vi "test-rotation3d.vi"(8 "error in (no error)":errorcluster) -> (0 "error out":errorcluster, 3 "ALL TESTS PASSED":bool)   [LabVIEW 2019]
uses:
  <vilib>/Rock Robotics/WPI/ThirdParty/JAS_Junk/TrajLib/Quaternion_New_Default.vi
  <vilib>/Rock Robotics/WPI/ThirdParty/JAS_Junk/TrajLib/Matrix_NormF.vi
  <vilib>/Rock Robotics/WPI/ThirdParty/JAS_Junk/TrajLib/Quaternion_New.vi
  <vilib>/Rock Robotics/WPI/ThirdParty/JAS_Junk/TrajLib/Rotation3d_Times.vi
  <vilib>/Rock Robotics/WPI/ThirdParty/JAS_Junk/TrajLib/MathUtil_Clamp.vi
  <vilib>/Rock Robotics/WPI/ThirdParty/JAS_Junk/TrajLib/Quaternion_Get_All.vi
  <vilib>/Rock Robotics/WPI/ThirdParty/JAS_Junk/TrajLib/Rotation3d_GetQuaterion.vi
  <vilib>/Rock Robotics/WPI/ThirdParty/JAS_Junk/TrajLib/Quaternion_Equals.vi
  <vilib>/Rock Robotics/WPI/ThirdParty/JAS_Junk/TrajLib/Util_CalcDist.vi
  <vilib>/Rock Robotics/WPI/ThirdParty/JAS_Junk/TrajLib/Quaternion_Get_Vect.vi
  <vilib>/Rock Robotics/WPI/ThirdParty/JAS_Junk/TrajLib/Quaternion_Get_W.vi
  <vilib>/Rock Robotics/WPI/ThirdParty/JAS_Junk/TrajLib/Rotation3d_UnaryMinus.vi
  <vilib>/Rock Robotics/WPI/ThirdParty/JAS_Junk/TrajLib/Rotation3d_Create_Quaternion.vi
  <vilib>/Rock Robotics/WPI/ThirdParty/JAS_Junk/TrajLib/Quaternion_Times.vi
  <vilib>/Analysis/_algsub.llb/Matrix Norm.vi
  <vilib>/Analysis/_algsub.llb/Real Matrix Norm.vi
  <vilib>/Rock Robotics/WPI/ThirdParty/JAS_Junk/TrajLib/Quaternion_Inverse.vi
  <vilib>/Rock Robotics/WPI/ThirdParty/JAS_Junk/TrajLib/Quaternion_Normalize.vi
  <vilib>/Rock Robotics/WPI/ThirdParty/JAS_Junk/TrajLib/Quaternion_Get_LVQuat.vi
  <vilib>/Rock Robotics/WPI/ThirdParty/JAS_Junk/TrajLib/Quaternion_New_LVQuat.vi
  <vilib>/Analysis/Matrix/Numeric/Conversions/Array To Matrix - RA.vi
  <vilib>/robotics/Kinematics/Multiply Quaternions.vi
  <vilib>/robotics/Kinematics/Multiply Quaternion by Quaternion.vi
  <vilib>/Rock Robotics/WPI/ThirdParty/JAS_Junk/TrajLib/Trajectory_Library.lvlib
  <vilib>/Analysis/Matrix/NI_Matrix.lvlib
panel:
  # "ROTATION3D TEST"
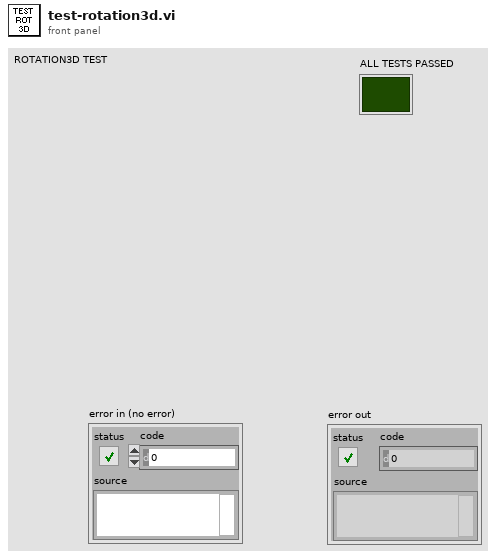
[diagram p1: front panel]
types:
  T1 = typedef "Trajectory_Library.lvlib/ROTATION3D.ctl" = cluster{"Q_quaternion":T2}
  T2 = typedef "Trajectory_Library.lvlib/QUATERNION.ctl" = cluster{"R":dbl, "V":dbl[]}
  T3 = typedef "Trajectory_Library.lvlib/ROTATION2D.ctl" = cluster{"VALUE":dbl, "COS":dbl, "SIN":dbl}
  T4 = typedef "NI_Matrix.lvlib/RealMatrix.ctl" = dbl[][]
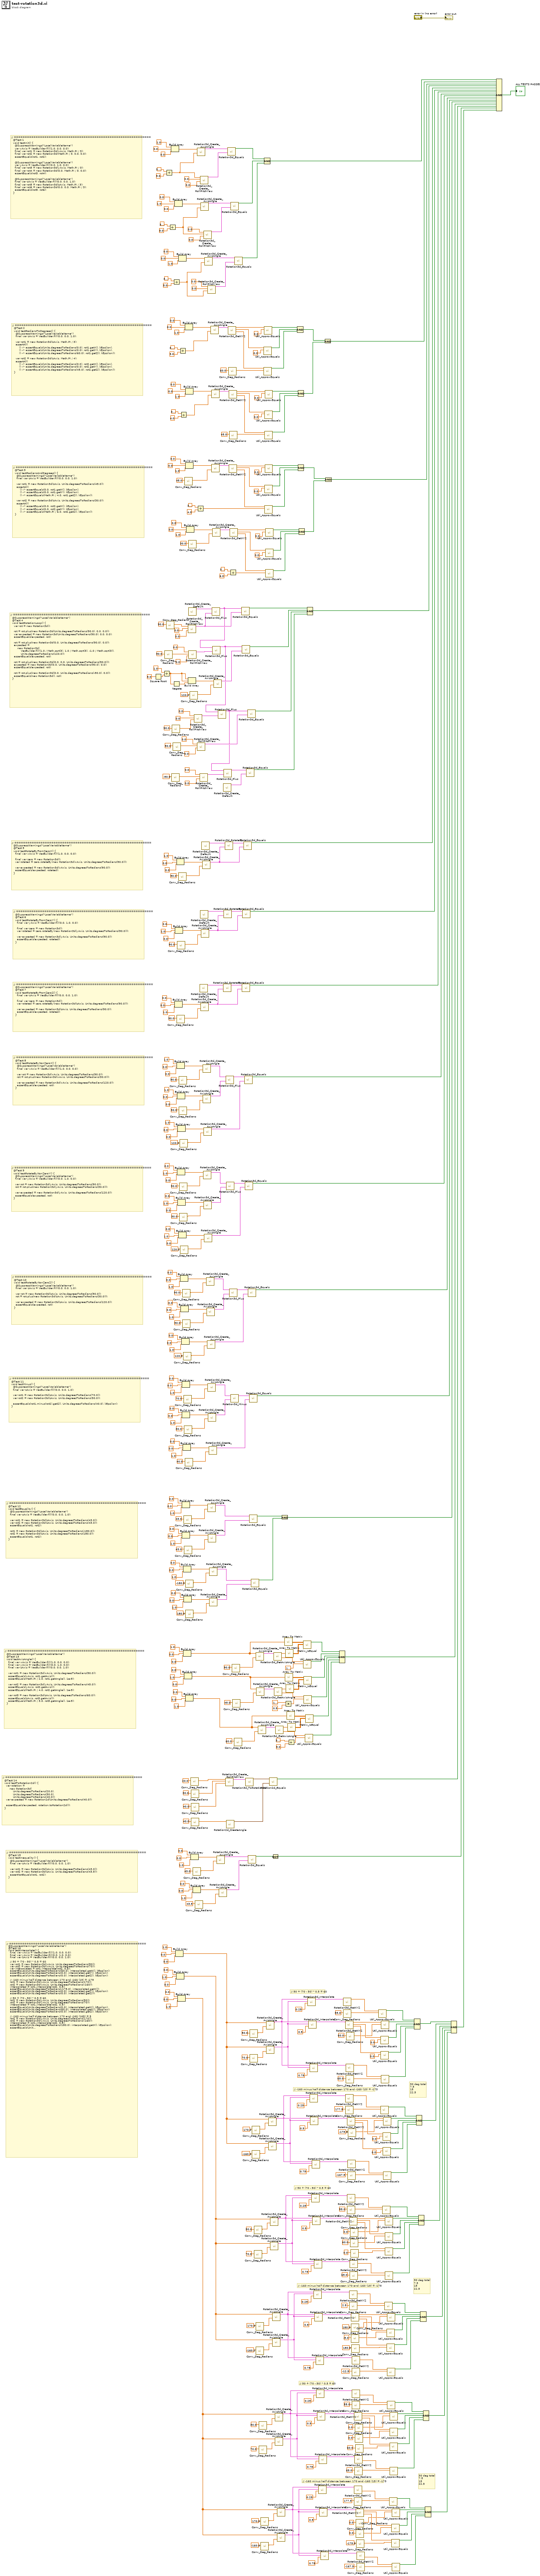
[diagram p0: block diagram]
diagram:
  # "30 deg total\n7.5\n15\n22.5"
  # "// -160 minus half distance between 170 and -160 (15) = -175"
  # "// 50 + (70 - 50) * 0.5 = 60"
  # "30 deg total\n7.5\n15\n22.5"
  # "// -160 minus half distance between 170 and -160 (15) = -175"
  # "// 50 + (70 - 50) * 0.5 = 60"
  # "30 deg total\n7.5\n15\n22.5"
  # "// -160 minus half distance between 170 and -160 (15) = -175"
  # "// 50 + (70 - 50) * 0.5 = 60"
  # "// ===============================================================\n  @SuppressWarnings(\"LocalVariableName\")\n  @Test 16\n  void testInterpolate() {\n    final var xAxis = VecBuilder.fill(1.0, 0.0, 0.0);\n    final var yAxis = VecBuilder.fill(0.0, 1.0, 0.0);\n    final var zAxis = VecBuilder.fill(0.0, 0.0, 1.0);\n\n    // 50 + (70 - 50) * 0.5 = 60\n    var rot1 = new Rotation3d(xAxis, Units.degreesToRadians(50));\n    var rot2 = new Rotation3d(xAxis, Units.degreesToRadians(70));\n    var interpolated = rot1.interpolate(rot2, 0.5);\n    assertEquals(Units.degreesToRadians(60.0), interpolated.getX(), kEpsilon);\n    assertEquals(Units.degreesToRadians(0.0), interpolated.getY(), kEpsilon);\n    assertEquals(Units.degreesToRadians(0.0), interpolated.getZ(), kEpsilon);\n\n    // -160 minus half distance between 170 and -160 (15) = -175\n    rot1 = new Rotation3d(xAxis, Units.degreesToRadians(170));\n    rot2 = new Rotation3d(xAxis, Units.degreesToRadians(-160));\n    interpolated = rot1.interpolate(rot2, 0.5);\n    assertEquals(Units.degreesToRadians(-175.0), interpolated.getX());\n    assertEquals(Units.degreesToRadians(0.0), interpolated.getY(), kEpsilon);\n    assertEquals(Units.degreesToRadians(0.0), interpolated.getZ());\n\n    // 50 + (70 - 50) * 0.5 = 60\n    rot1 = new Rotation3d(yAxis, Units.degreesToRadians(50));\n    rot2 = new Rotation3d(yAxis, Units.degreesToRadians(70));\n    interpolated = rot1.interpolate(rot2, 0.5);\n    assertEquals(Units.degreesToRadians(0.0), interpolated.getX(), kEpsilon);\n    assertEquals(Units.degreesToRadians(60.0), interpolated.getY(), kEpsilon);\n    assertEquals(Units.degreesToRadians(0.0), interpolated.getZ(), kEpsilon);\n\n    // -160 minus half distance between 170 and -160 (165) = 5\n    rot1 = new Rotation3d(yAxis, Units.degreesToRadians(170));\n    rot2 = new Rotation3d(yAxis, Units.degreesToRadians(-160));\n    interpolated = rot1.interpolate(rot2, 0.5);\n    assertEquals(Units.degreesToRadians(180.0), interpolated.getX(), kEpsilon);\n    assertEquals(Units.degreesToRadians(-5.0), interpolated.getY(), kEpsilon);\n    assertEquals(Units.degreesToRadians(180.0), interpolated.getZ(), kEpsilon);\n\n    // 50 + (70 - 50) * 0.5 = 60\n    rot1 = new Rotation3d(zAxis, Units.degreesToRadians(50));\n    rot2 = new Rotation3d(zAxis, Units.degreesToRadians(70));\n    interpolated = rot1.interpolate(rot2, 0.5);\n    assertEquals(Units.degreesToRadians(0.0), interpolated.getX(), kEpsilon);\n    assertEquals(Units.degreesToRadians(0.0), interpolated.getY(), kEpsilon);\n    assertEquals(Units.degreesToRadians(60.0), interpolated.getZ(), kEpsilon);\n\n    // -160 minus half distance between 170 and -160 (15) = -175\n    rot1 = new Rotation3d(zAxis, Units.degreesToRadians(170));\n    rot2 = new Rotation3d(zAxis, Units.degreesToRadians(-160));\n    interpolated = rot1.interpolate(rot2, 0.5);\n    assertEquals(Units.degreesToRadians(0.0), interpolated.getX(), kEpsilon);\n    assertEquals(Units.degreesToRadians(0.0), interpolated.getY(), kEpsilon);\n    assertEquals(Units.degreesToRadians(-175.0), interpolated.getZ(), kEpsilon);\n  }"
  # "// ===============================================================\n  @Test 15\n  void testInequality() {\n    @SuppressWarnings(\"LocalVariableName\")\n    final var zAxis = VecBuilder.fill(0.0, 0.0, 1.0);\n\n    var rot1 = new Rotation3d(zAxis, Units.degreesToRadians(43.0));\n    var rot2 = new Rotation3d(zAxis, Units.degreesToRadians(43.5));\n    assertNotEquals(rot1, rot2);\n  }"
  # "// ===============================================================\n  @Test 14\n  void testToRotation2d() {\n    var rotation =\n        new Rotation3d(\n            Units.degreesToRadians(20.0),\n            Units.degreesToRadians(30.0),\n            Units.degreesToRadians(40.0));\n    var expected = new Rotation2d(Units.degreesToRadians(40.0));\n\n    assertEquals(expected, rotation.toRotation2d());\n  }"
  # "// ===============================================================\n  @SuppressWarnings(\"LocalVariableName\")\n  @Test 13\n  void testAxisAngle() {\n    final var xAxis = VecBuilder.fill(1.0, 0.0, 0.0);\n    final var yAxis = VecBuilder.fill(0.0, 1.0, 0.0);\n    final var zAxis = VecBuilder.fill(0.0, 0.0, 1.0);\n\n    var rot1 = new Rotation3d(xAxis, Units.degreesToRadians(90.0));\n    assertEquals(xAxis, rot1.getAxis());\n    assertEquals(Math.PI / 2.0, rot1.getAngle(), 1e-9);\n\n    var rot2 = new Rotation3d(yAxis, Units.degreesToRadians(45.0));\n    assertEquals(yAxis, rot2.getAxis());\n    assertEquals(Math.PI / 4.0, rot2.getAngle(), 1e-9);\n\n    var rot3 = new Rotation3d(zAxis, Units.degreesToRadians(60.0));\n    assertEquals(zAxis, rot3.getAxis());\n    assertEquals(Math.PI / 3.0, rot3.getAngle(), 1e-9);\n  }"
  # "// ===============================================================\n  @Test 12\n  void testEquality() {\n    @SuppressWarnings(\"LocalVariableName\")\n    final var zAxis = VecBuilder.fill(0.0, 0.0, 1.0);\n\n    var rot1 = new Rotation3d(zAxis, Units.degreesToRadians(43.0));\n    var rot2 = new Rotation3d(zAxis, Units.degreesToRadians(43.0));\n    assertEquals(rot1, rot2);\n\n    rot1 = new Rotation3d(zAxis, Units.degreesToRadians(-180.0));\n    rot2 = new Rotation3d(zAxis, Units.degreesToRadians(180.0));\n    assertEquals(rot1, rot2);\n  }"
  # "// ===============================================================\n  @Test 11\n  void testMinus() {\n    @SuppressWarnings(\"LocalVariableName\")\n    final var zAxis = VecBuilder.fill(0.0, 0.0, 1.0);\n\n    var rot1 = new Rotation3d(zAxis, Units.degreesToRadians(70.0));\n    var rot2 = new Rotation3d(zAxis, Units.degreesToRadians(30.0));\n\n    assertEquals(rot1.minus(rot2).getZ(), Units.degreesToRadians(40.0), kEpsilon);\n  }"
  # "// ===============================================================\n  @Test 10\n  void testRotateByNonZeroZ() {\n    @SuppressWarnings(\"LocalVariableName\")\n    final var zAxis = VecBuilder.fill(0.0, 0.0, 1.0);\n\n    var rot = new Rotation3d(zAxis, Units.degreesToRadians(90.0));\n    rot = rot.plus(new Rotation3d(zAxis, Units.degreesToRadians(30.0)));\n\n    var expected = new Rotation3d(zAxis, Units.degreesToRadians(120.0));\n    assertEquals(expected, rot);\n  }"
  # "// ===============================================================\n  @Test 9\n  void testRotateByNonZeroY() {\n    @SuppressWarnings(\"LocalVariableName\")\n    final var yAxis = VecBuilder.fill(0.0, 1.0, 0.0);\n\n    var rot = new Rotation3d(yAxis, Units.degreesToRadians(90.0));\n    rot = rot.plus(new Rotation3d(yAxis, Units.degreesToRadians(30.0)));\n\n    var expected = new Rotation3d(yAxis, Units.degreesToRadians(120.0));\n    assertEquals(expected, rot);\n  }"
  # "// ===============================================================\n  @Test 8\n  void testRotateByNonZeroX() {\n    @SuppressWarnings(\"LocalVariableName\")\n    final var xAxis = VecBuilder.fill(1.0, 0.0, 0.0);\n\n    var rot = new Rotation3d(xAxis, Units.degreesToRadians(90.0));\n    rot = rot.plus(new Rotation3d(xAxis, Units.degreesToRadians(30.0)));\n\n    var expected = new Rotation3d(xAxis, Units.degreesToRadians(120.0));\n    assertEquals(expected, rot);\n  }"
  # "// ===============================================================\n  @SuppressWarnings(\"LocalVariableName\")\n  @Test 7\n  void testRotateByFromZeroZ() {\n    final var zAxis = VecBuilder.fill(0.0, 0.0, 1.0);\n\n    final var zero = new Rotation3d();\n    var rotated = zero.rotateBy(new Rotation3d(zAxis, Units.degreesToRadians(90.0)));\n\n    var expected = new Rotation3d(zAxis, Units.degreesToRadians(90.0));\n    assertEquals(expected, rotated);\n  }"
  # "// ===============================================================\n  @SuppressWarnings(\"LocalVariableName\")\n  @Test 6\n  void testRotateByFromZeroY() {\n    final var yAxis = VecBuilder.fill(0.0, 1.0, 0.0);\n\n    final var zero = new Rotation3d();\n    var rotated = zero.rotateBy(new Rotation3d(yAxis, Units.degreesToRadians(90.0)));\n\n    var expected = new Rotation3d(yAxis, Units.degreesToRadians(90.0));\n    assertEquals(expected, rotated);\n  }"
  # "// ===============================================================\n  @SuppressWarnings(\"LocalVariableName\")\n  @Test 5\n  void testRotateByFromZeroX() {\n    final var xAxis = VecBuilder.fill(1.0, 0.0, 0.0);\n\n    final var zero = new Rotation3d();\n    var rotated = zero.rotateBy(new Rotation3d(xAxis, Units.degreesToRadians(90.0)));\n\n    var expected = new Rotation3d(xAxis, Units.degreesToRadians(90.0));\n    assertEquals(expected, rotated);\n  }"
  # "// ===============================================================\n  @SuppressWarnings(\"LocalVariableName\")\n  @Test 4\n  void testRotationLoop() {\n    var rot = new Rotation3d();\n\n    rot = rot.plus(new Rotation3d(Units.degreesToRadians(90.0), 0.0, 0.0));\n    var expected = new Rotation3d(Units.degreesToRadians(90.0), 0.0, 0.0);\n    assertEquals(expected, rot);\n\n    rot = rot.plus(new Rotation3d(0.0, Units.degreesToRadians(90.0), 0.0));\n    expected =\n        new Rotation3d(\n            VecBuilder.fill(1.0 / Math.sqrt(3), 1.0 / Math.sqrt(3), -1.0 / Math.sqrt(3)),\n            Units.degreesToRadians(120.0));\n    assertEquals(expected, rot);\n\n    rot = rot.plus(new Rotation3d(0.0, 0.0, Units.degreesToRadians(90.0)));\n    expected = new Rotation3d(0.0, Units.degreesToRadians(90.0), 0.0);\n    assertEquals(expected, rot);\n\n    rot = rot.plus(new Rotation3d(0.0, Units.degreesToRadians(-90.0), 0.0));\n    assertEquals(new Rotation3d(), rot);\n  }"
  # "// ===============================================================\n  @Test 3\n  void testRadiansAndDegrees() {\n    @SuppressWarnings(\"LocalVariableName\")\n    final var zAxis = VecBuilder.fill(0.0, 0.0, 1.0);\n\n    var rot1 = new Rotation3d(zAxis, Units.degreesToRadians(45.0));\n    assertAll(\n        () -> assertEquals(0.0, rot1.getX(), kEpsilon),\n        () -> assertEquals(0.0, rot1.getY(), kEpsilon),\n        () -> assertEquals(Math.PI / 4.0, rot1.getZ(), kEpsilon));\n\n    var rot2 = new Rotation3d(zAxis, Units.degreesToRadians(30.0));\n    assertAll(\n        () -> assertEquals(0.0, rot2.getX(), kEpsilon),\n        () -> assertEquals(0.0, rot2.getY(), kEpsilon),\n        () -> assertEquals(Math.PI / 6.0, rot2.getZ(), kEpsilon));\n  }"
  # "// ===============================================================\n  @Test 2\n  void testRadiansToDegrees() {\n    @SuppressWarnings(\"LocalVariableName\")\n    final var zAxis = VecBuilder.fill(0.0, 0.0, 1.0);\n\n    var rot1 = new Rotation3d(zAxis, Math.PI / 3);\n    assertAll(\n        () -> assertEquals(Units.degreesToRadians(0.0), rot1.getX(), kEpsilon),\n        () -> assertEquals(Units.degreesToRadians(0.0), rot1.getY(), kEpsilon),\n        () -> assertEquals(Units.degreesToRadians(60.0), rot1.getZ(), kEpsilon));\n\n    var rot2 = new Rotation3d(zAxis, Math.PI / 4);\n    assertAll(\n        () -> assertEquals(Units.degreesToRadians(0.0), rot2.getX(), kEpsilon),\n        () -> assertEquals(Units.degreesToRadians(0.0), rot2.getY(), kEpsilon),\n        () -> assertEquals(Units.degreesToRadians(45.0), rot2.getZ(), kEpsilon));\n  }"
  # "// ===============================================================\n  @Test 1\n  void testInit() {\n    @SuppressWarnings(\"LocalVariableName\")\n    var xAxis = VecBuilder.fill(1.0, 0.0, 0.0);\n    final var rot1 = new Rotation3d(xAxis, Math.PI / 3);\n    final var rot2 = new Rotation3d(Math.PI / 3, 0.0, 0.0);\n    assertEquals(rot1, rot2);\n\n    @SuppressWarnings(\"LocalVariableName\")\n    var yAxis = VecBuilder.fill(0.0, 1.0, 0.0);\n    final var rot3 = new Rotation3d(yAxis, Math.PI / 3);\n    final var rot4 = new Rotation3d(0.0, Math.PI / 3, 0.0);\n    assertEquals(rot3, rot4);\n\n    @SuppressWarnings(\"LocalVariableName\")\n    final var zAxis = VecBuilder.fill(0.0, 0.0, 1.0);\n    final var rot5 = new Rotation3d(zAxis, Math.PI / 3);\n    final var rot6 = new Rotation3d(0.0, 0.0, Math.PI / 3);\n    assertEquals(rot5, rot6);\n  }"
  n1 = Square Root(x=3.0) -> (sqrt(x)=w462:dbl)
  n2 = Divide(x=1.0, y=w462) -> (x/y=w459:dbl)
  n3 = call <vilib>:"Conv_Deg_Radians.vi"("Degress"=90.0) -> ("Radians"=w469:dbl)  [unwired: 10 in]
  n4 = Divide(x=3.141592653589793, y=3.0) -> (x/y=w587:dbl)
  n5 = call <vilib>:"Conv_Deg_Radians.vi"("Degress"=90.0) -> ("Radians"=w479:dbl)  [unwired: 10 in]
  n6 = Divide(x=3.141592653589793, y=3.0) -> (x/y=w562:dbl)
  n7 = Build Array(1.0 ("element"), 0.0 ("element"), 0.0 ("element")) -> (w592:dbl[])
  n8 = call <vilib>:"Conv_Deg_Radians.vi"("Degress"=-90.0) -> ("Radians"=w440:dbl)  [unwired: 10 in]
  n9 = call <vilib>:"Conv_Deg_Radians.vi"("Degress"=90.0) -> ("Radians"=w452:dbl)  [unwired: 10 in]
  n10 = Divide(x=3.141592653589793, y=3.0) -> (x/y=w559:dbl)
  n11 = Negate(x=w459) -> (-x=w460:dbl)
  n12 = call <vilib>:"Conv_Deg_Radians.vi"("Degress"=90.0) -> ("Radians"=w448:dbl)  [unwired: 10 in]
  n13 = Build Array(0.0 ("element"), 1.0 ("element"), 0.0 ("element")) -> (w581:dbl[])
  n14 = Build Array(0.0 ("element"), 0.0 ("element"), 1.0 ("element")) -> (w415:dbl[])
  n15 = Build Array(0.0 ("element"), 1.0 ("element"), 0.0 ("element")) -> (w425:dbl[])
  n16 = Build Array(1.0 ("element"), 0.0 ("element"), 0.0 ("element")) -> (w140:dbl[])
  n17 = Build Array(0.0 ("element"), 1.0 ("element"), 0.0 ("element")) -> (w89:dbl[])
  n18 = Build Array(1.0 ("element"), 0.0 ("element"), 0.0 ("element")) -> (w435:dbl[])
  n19 = call <vilib>:"Conv_Deg_Radians.vi"("Degress"=90.0) -> ("Radians"=w413:dbl)  [unwired: 10 in]
  n20 = Build Array(1.0 ("element"), 0.0 ("element"), 0.0 ("element")) -> (w397:dbl[])
  n21 = call <vilib>:"Conv_Deg_Radians.vi"("Degress"=90.0) -> ("Radians"=w423:dbl)  [unwired: 10 in]
  n22 = Build Array(1.0 ("element"), 0.0 ("element"), 0.0 ("element")) -> (w405:dbl[])
  n23 = Build Array(0.0 ("element"), 1.0 ("element"), 0.0 ("element")) -> (w374:dbl[])
  n24 = Build Array(0.0 ("element"), 1.0 ("element"), 0.0 ("element")) -> (w382:dbl[])
  n25 = Build Array(1.0 ("element"), 0.0 ("element"), 0.0 ("element")) -> (w390:dbl[])
  n26 = Build Array(0.0 ("element"), 0.0 ("element"), 1.0 ("element")) -> (w12:dbl[])
  n27 = Build Array(0.0 ("element"), 1.0 ("element"), 0.0 ("element")) -> (w367:dbl[])
  n28 = Build Array(0.0 ("element"), 0.0 ("element"), 1.0 ("element")) -> (w572:dbl[])
  n29 = call <vilib>:"Conv_Deg_Radians.vi"("Degress"=90.0) -> ("Radians"=w433:dbl)  [unwired: 10 in]
  n30 = call <vilib>:"Conv_Deg_Radians.vi"("Degress"=90.0) -> ("Radians"=w395:dbl)  [unwired: 10 in]
  n31 = Divide(x=3.141592653589793, y=3.0) -> (x/y=w552:dbl)
  n32 = call <vilib>:"Conv_Deg_Radians.vi"("Degress"=30.0) -> ("Radians"=w403:dbl)  [unwired: 10 in]
  n33 = call <vilib>:"Conv_Deg_Radians.vi"("Degress"=90.0) -> ("Radians"=w372:dbl)  [unwired: 10 in]
  n34 = call <vilib>:"Conv_Deg_Radians.vi"("Degress"=30.0) -> ("Radians"=w380:dbl)  [unwired: 10 in]
  n35 = Divide(x=3.141592653589793, y=4.0) -> (x/y=w533:dbl)
  n36 = call <vilib>:"Conv_Deg_Radians.vi"("Degress"=120.0) -> ("Radians"=w388:dbl)  [unwired: 10 in]
  n37 = call <vilib>:"Conv_Deg_Radians.vi"("Degress"=120.0) -> ("Radians"=w365:dbl)  [unwired: 10 in]
  n38 = Build Array(0.0 ("element"), 0.0 ("element"), 1.0 ("element")) -> (w351:dbl[])
  n39 = Build Array(0.0 ("element"), 0.0 ("element"), 1.0 ("element")) -> (w359:dbl[])
  n40 = Build Array(0.0 ("element"), 0.0 ("element"), 1.0 ("element")) -> (w344:dbl[])
  n41 = Build Array(0.0 ("element"), 0.0 ("element"), 1.0 ("element")) -> (w328:dbl[])
  n42 = Build Array(0.0 ("element"), 0.0 ("element"), 1.0 ("element")) -> (w307:dbl[])
  n43 = Build Array(0.0 ("element"), 0.0 ("element"), 1.0 ("element")) -> (w336:dbl[])
  n44 = Build Array(0.0 ("element"), 0.0 ("element"), 1.0 ("element")) -> (w313:dbl[])
  n45 = call <vilib>:"Conv_Deg_Radians.vi"("Degress"=90.0) -> ("Radians"=w349:dbl)  [unwired: 10 in]
  n46 = call <vilib>:"Conv_Deg_Radians.vi"("Degress"=30.0) -> ("Radians"=w357:dbl)  [unwired: 10 in]
  n47 = Build Array(0.0 ("element"), 0.0 ("element"), 1.0 ("element")) -> (w321:dbl[])
  n48 = Build Array(1.0 ("element"), 0.0 ("element"), 0.0 ("element")) -> (w269:dbl[])
  n49 = call <vilib>:"Conv_Deg_Radians.vi"("Degress"=120.0) -> ("Radians"=w342:dbl)  [unwired: 10 in]
  n50 = Build Array(0.0 ("element"), 0.0 ("element"), 1.0 ("element")) -> (w293:dbl[])
  n51 = Build Array(0.0 ("element"), 0.0 ("element"), 1.0 ("element")) -> (w299:dbl[])
  n52 = call <vilib>:"Conv_Deg_Radians.vi"("Degress"=70.0) -> ("Radians"=w326:dbl)  [unwired: 10 in]
  n53 = call <vilib>:"Conv_Deg_Radians.vi"("Degress"=43.0) -> ("Radians"=w305:dbl)  [unwired: 10 in]
  n54 = call <vilib>:"Conv_Deg_Radians.vi"("Degress"=30.0) -> ("Radians"=w334:dbl)  [unwired: 10 in]
  n55 = call <vilib>:"Conv_Deg_Radians.vi"("Degress"=43.0) -> ("Radians"=w311:dbl)  [unwired: 10 in]
  n56 = Build Array(0.0 ("element"), 1.0 ("element"), 0.0 ("element")) -> (w248:dbl[])
  n57 = call <vilib>:"Conv_Deg_Radians.vi"("Degress"=45.0) -> ("Radians"=w490:dbl)  [unwired: 10 in]
  n58 = Build Array(0.0 ("element"), 0.0 ("element"), 1.0 ("element")) -> (w555:dbl[])
  n59 = call <vilib>:"Conv_Deg_Radians.vi"("Degress"=40.0) -> ("Radians"=w319:dbl)  [unwired: 10 in]
  n60 = call <vilib>:"Conv_Deg_Radians.vi"("Degress"=-180.0) -> ("Radians"=w291:dbl)  [unwired: 10 in]
  n61 = Build Array(0.0 ("element"), 0.0 ("element"), 1.0 ("element")) -> (w536:dbl[])
  n62 = Build Array(0.0 ("element"), 0.0 ("element"), 1.0 ("element")) -> (w516:dbl[])
  n63 = call <vilib>:"Conv_Deg_Radians.vi"("Degress"=180.0) -> ("Radians"=w297:dbl)  [unwired: 10 in]
  n64 = Build Array(0.0 ("element"), 0.0 ("element"), 1.0 ("element")) -> (w247:dbl[])
  n65 = Build Array(0.0 ("element"), 0.0 ("element"), 1.0 ("element")) -> (w502:dbl[])
  n66 = Build Array(w459, w459, w460) -> (w467:dbl[])
  n67 = call <vilib>:"Rotation3d_Create_RollPitchYaw.vi"("Yaw"=0.0, "Pitch"=0.0, "Roll"=w479) -> ("Rotation3d"=w475:T1)  [unwired: 8 in]
  n68 = call <vilib>:"Conv_Deg_Radians.vi"("Degress"=30.0) -> ("Radians"=w485:dbl)  [unwired: 10 in]
  n69 = call <vilib>:"Rotation3d_Create_Default.vi"() -> ("ROTATION3D"=w476:T1)  [unwired: 11 in]
  n70 = call <vilib>:"Rotation3d_Create_RollPitchYaw.vi"("Yaw"=0.0, "Pitch"=w469, "Roll"=0.0 ("Pitch")) -> ("Rotation3d"=w471:T1)  [unwired: 8 in]
  n71 = call <vilib>:"Conv_Deg_Radians.vi"("Degress"=120.0) -> ("Radians"=w465:dbl)  [unwired: 10 in]
  n72 = call <vilib>:"Conv_Deg_Radians.vi"("Degress"=20.0) -> ("Radians"=w232:dbl)  [unwired: 10 in]
  n73 = Build Array(0.0 ("element"), 0.0 ("element"), 1.0 ("element")) -> (w223:dbl[])
  n74 = call <vilib>:"Conv_Deg_Radians.vi"("Degress"=30.0) -> ("Radians"=w231:dbl)  [unwired: 10 in]
  n75 = call <vilib>:"Conv_Deg_Radians.vi"("Degress"=40.0) -> ("Radians"=w230:dbl)  [unwired: 10 in]
  n76 = call <vilib>:"Conv_Deg_Radians.vi"("Degress"=40.0) -> ("Radians"=w228:dbl)  [unwired: 10 in]
  n77 = call <vilib>:"Conv_Deg_Radians.vi"("Degress"=43.0) -> ("Radians"=w221:dbl)  [unwired: 10 in]
  n78 = Build Array(0.0 ("element"), 0.0 ("element"), 1.0 ("element")) -> (w217:dbl[])
  n79 = call <vilib>:"Rotation3d_Create_RollPitchYaw.vi"("Yaw"=w452, "Pitch"=0.0 ("Yaw"), "Roll"=0.0 ("Pitch")) -> ("Rotation3d"=w456:T1)  [unwired: 8 in]
  n80 = call <vilib>:"Conv_Deg_Radians.vi"("Degress"=43.5) -> ("Radians"=w215:dbl)  [unwired: 10 in]
  n81 = Divide(x=3.141592653589793, y=4.0) -> (x/y=w487:dbl)
  n82 = call <vilib>:"Rotation3d_Create_AxisAngle.vi"("Angle"=w587, "Axis Vector"=w592) -> ("Rotation3d"=w586:T1)  [unwired: 9 in]
  n83 = call <vilib>:"Rotation3d_Create_RollPitchYaw.vi"("Yaw"=0.0, "Pitch"=w448, "Roll"=0.0 ("Pitch")) -> ("Rotation3d"=w447:T1)  [unwired: 8 in]
  n84 = call <vilib>:"Rotation3d_Create_RollPitchYaw.vi"("Yaw"=0.0, "Pitch"=w440, "Roll"=0.0 ("Pitch")) -> ("Rotation3d"=w444:T1)  [unwired: 8 in]
  n85 = call <vilib>:"Rotation3d_Create_Default.vi"() -> ("ROTATION3D"=w408:T1)  [unwired: 11 in]
  n86 = call <vilib>:"Rotation3d_Create_RollPitchYaw.vi"("Yaw"=0.0, "Pitch"=0.0, "Roll"=w587) -> ("Rotation3d"=w585:T1)  [unwired: 8 in]
  n87 = call <vilib>:"Rotation3d_Create_Default.vi"() -> ("ROTATION3D"=w418:T1)  [unwired: 11 in]
  n88 = call <vilib>:"Rotation3d_Create_AxisAngle.vi"("Angle"=w562, "Axis Vector"=w581) -> ("Rotation3d"=w577:T1)  [unwired: 9 in]
  n89 = call <vilib>:"Rotation3d_Create_AxisAngle.vi"("Angle"=w413, "Axis Vector"=w415) -> ("Rotation3d"=w407:T1)  [unwired: 9 in]
  n90 = call <vilib>:"Rotation3d_Create_AxisAngle.vi"("Angle"=w423, "Axis Vector"=w425) -> ("Rotation3d"=w417:T1)  [unwired: 9 in]
  n91 = call <vilib>:"Rotation3d_Create_Default.vi"() -> ("ROTATION3D"=w429:T1)  [unwired: 11 in]
  n92 = call <vilib>:"Rotation3d_Create_AxisAngle.vi"("Angle"=w433, "Axis Vector"=w435) -> ("Rotation3d"=w427:T1)  [unwired: 9 in]
  n93 = call <vilib>:"Rotation3d_Create_AxisAngle.vi"("Angle"=w395, "Axis Vector"=w397) -> ("Rotation3d"=w391:T1)  [unwired: 9 in]
  n94 = call <vilib>:"Rotation3d_Create_AxisAngle.vi"("Angle"=w403, "Axis Vector"=w405) -> ("Rotation3d"=w398:T1)  [unwired: 9 in]
  n95 = call <vilib>:"Rotation3d_Create_AxisAngle.vi"("Angle"=w372, "Axis Vector"=w374) -> ("Rotation3d"=w368:T1)  [unwired: 9 in]
  n96 = call <vilib>:"Rotation3d_Create_RollPitchYaw.vi"("Yaw"=0.0, "Pitch"=w562, "Roll"=0.0 ("Pitch")) -> ("Rotation3d"=w576:T1)  [unwired: 8 in]
  n97 = call <vilib>:"Rotation3d_Create_AxisAngle.vi"("Angle"=w380, "Axis Vector"=w382) -> ("Rotation3d"=w375:T1)  [unwired: 9 in]
  n98 = call <vilib>:"Rotation3d_Create_AxisAngle.vi"("Angle"=w388, "Axis Vector"=w390) -> ("Rotation3d"=w384:T1)  [unwired: 9 in]
  n99 = call <vilib>:"Rotation3d_Create_AxisAngle.vi"("Angle"=w365, "Axis Vector"=w367) -> ("Rotation3d"=w361:T1)  [unwired: 9 in]
  n100 = call <vilib>:"Rotation3d_Create_AxisAngle.vi"("Angle"=w559, "Axis Vector"=w572) -> ("Rotation3d"=w568:T1)  [unwired: 9 in]
  n101 = call <vilib>:"Rotation3d_Create_AxisAngle.vi"("Angle"=w349, "Axis Vector"=w351) -> ("Rotation3d"=w345:T1)  [unwired: 9 in]
  n102 = call <vilib>:"Rotation3d_Create_AxisAngle.vi"("Angle"=w357, "Axis Vector"=w359) -> ("Rotation3d"=w352:T1)  [unwired: 9 in]
  n103 = call <vilib>:"Rotation3d_Create_AxisAngle.vi"("Angle"=w342, "Axis Vector"=w344) -> ("Rotation3d"=w338:T1)  [unwired: 9 in]
  n104 = call <vilib>:"Rotation3d_Create_RollPitchYaw.vi"("Yaw"=w559, "Pitch"=0.0, "Roll"=0.0 ("Yaw")) -> ("Rotation3d"=w567:T1)  [unwired: 8 in]
  n105 = call <vilib>:"Rotation3d_Create_AxisAngle.vi"("Angle"=w326, "Axis Vector"=w328) -> ("Rotation3d"=w322:T1)  [unwired: 9 in]
  n106 = call <vilib>:"Rotation3d_Create_AxisAngle.vi"("Angle"=w305, "Axis Vector"=w307) -> ("Rotation3d"=w300:T1)  [unwired: 9 in]
  n107 = call <vilib>:"Rotation3d_Create_AxisAngle.vi"("Angle"=w334, "Axis Vector"=w336) -> ("Rotation3d"=w329:T1)  [unwired: 9 in]
  n108 = call <vilib>:"Rotation3d_Create_AxisAngle.vi"("Angle"=w311, "Axis Vector"=w313) -> ("Rotation3d"=w301:T1)  [unwired: 9 in]
  n109 = call <vilib>:"Rotation3d_Create_AxisAngle.vi"("Angle"=w319, "Axis Vector"=w321) -> ("Rotation3d"=w315:T1)  [unwired: 9 in]
  n110 = call <vilib>:"Rotation3d_Create_AxisAngle.vi"("Angle"=w291, "Axis Vector"=w293) -> ("Rotation3d"=w286:T1)  [unwired: 9 in]
  n111 = call <vilib>:"Rotation3d_Create_AxisAngle.vi"("Angle"=w297, "Axis Vector"=w299) -> ("Rotation3d"=w287:T1)  [unwired: 9 in]
  n112 = call <vilib>:"Rotation3d_Create_AxisAngle.vi"("Angle"=w552, "Axis Vector"=w555) -> ("Rotation3d"=w551:T1)  [unwired: 9 in]
  n113 = call <vilib>:"Rotation3d_Create_AxisAngle.vi"("Angle"=w533, "Axis Vector"=w536) -> ("Rotation3d"=w532:T1)  [unwired: 9 in]
  n114 = call <vilib>:"Rotation3d_Create_AxisAngle.vi"("Angle"=w490, "Axis Vector"=w516) -> ("Rotation3d"=w515:T1)  [unwired: 9 in]
  n115 = call <vilib>:"Rotation3d_Plus.vi"("other Rotation3d"=w475, "in Rotation3d"=w476) -> ("out Rotation3d"=w468:T1)  [unwired: 9 in]
  n116 = call <vilib>:"Rotation3d_Create_AxisAngle.vi"("Angle"=w485, "Axis Vector"=w502) -> ("Rotation3d"=w501:T1)  [unwired: 9 in]
  n117 = call <vilib>:"Rotation3d_Plus.vi"("other Rotation3d"=w471, "in Rotation3d"=w468) -> ("out Rotation3d"=w454:T1)  [unwired: 9 in]
  n118 = call <vilib>:"Rotation3d_Create_AxisAngle.vi"("Angle"=w465, "Axis Vector"=w467) -> ("Rotation3d"=w464:T1)  [unwired: 9 in]
  n119 = call <vilib>:"Rotation3d_Create_AxisAngle.vi"("Angle"=w221, "Axis Vector"=w223) -> ("Rotation3d"=w211:T1)  [unwired: 9 in]
  n120 = call <vilib>:"Rotation3d_Plus.vi"("other Rotation3d"=w456, "in Rotation3d"=w454) -> ("out Rotation3d"=w442:T1)  [unwired: 9 in]
  n121 = call <vilib>:"Rotation3d_Create_AxisAngle.vi"("Angle"=w215, "Axis Vector"=w217) -> ("Rotation3d"=w210:T1)  [unwired: 9 in]
  n122 = call <vilib>:"Rotation3d_Create_Default.vi"() -> ("ROTATION3D"=w438:T1)  [unwired: 11 in]
  n123 = call <vilib>:"Rotation3d_RotateBy.vi"("other Rotation3d"=w407, "in Rotation3d"=w408) -> ("out Rotation3d"=w409:T1)  [unwired: 9 in]
  n124 = call <vilib>:"Rotation3d_Plus.vi"("other Rotation3d"=w444, "in Rotation3d"=w442) -> ("out Rotation3d"=w439:T1)  [unwired: 9 in]
  n125 = call <vilib>:"Rotation3d_RotateBy.vi"("other Rotation3d"=w417, "in Rotation3d"=w418) -> ("out Rotation3d"=w419:T1)  [unwired: 9 in]
  n126 = call <vilib>:"Rotation3d_RotateBy.vi"("other Rotation3d"=w427, "in Rotation3d"=w429) -> ("out Rotation3d"=w428:T1)  [unwired: 9 in]
  n127 = call <vilib>:"Rotation3d_Create_RollPitchYaw.vi"("Yaw"=w230, "Pitch"=w231, "Roll"=w232) -> ("Rotation3d"=w227:T1)  [unwired: 8 in]
  n128 = call <vilib>:"Rotation3d_Plus.vi"("other Rotation3d"=w398, "in Rotation3d"=w391) -> ("out Rotation3d"=w399:T1)  [unwired: 9 in]
  n129 = call <vilib>:"Rotation3d_Plus.vi"("other Rotation3d"=w375, "in Rotation3d"=w368) -> ("out Rotation3d"=w376:T1)  [unwired: 9 in]
  n130 = call <vilib>:"Rotation2d_CreateAngle.vi"("Angle"=w228) -> ("ROTATION"=w225:T3)  [unwired: 10 in]
  n131 = call <vilib>:"Rotation3d_Equals.vi"("other Rotation3d"=w585, "in Rotation3d"=w586) -> ("Equals"=w566:bool)  [unwired: 9 in]
  n132 = call <vilib>:"Rotation3d_GetXYZ.vi"("in Rotation3d"=w551) -> ("Z"=w543:dbl, "Y"=w544:dbl, "X"=w545:dbl)  [unwired: 8 in]
  n133 = call <vilib>:"Conv_Deg_Radians.vi"("Degress"=60.0) -> ("Radians"=w541:dbl)  [unwired: 10 in]
  n134 = call <vilib>:"Rotation3d_GetXYZ.vi"("in Rotation3d"=w532) -> ("Z"=w524:dbl, "Y"=w525:dbl, "X"=w526:dbl)  [unwired: 8 in]
  n135 = call <vilib>:"Rotation3d_GetXYZ.vi"("in Rotation3d"=w515) -> ("Z"=w507:dbl, "Y"=w508:dbl, "X"=w509:dbl)  [unwired: 8 in]
  n136 = call <vilib>:"Conv_Deg_Radians.vi"("Degress"=45.0) -> ("Radians"=w522:dbl)  [unwired: 10 in]
  n137 = Divide(x=3.141592653589793, y=6.0) -> (x/y=w482:dbl)
  n138 = call <vilib>:"Rotation3d_Plus.vi"("other Rotation3d"=w352, "in Rotation3d"=w345) -> ("out Rotation3d"=w353:T1)  [unwired: 9 in]
  n139 = call <vilib>:"Rotation3d_GetXYZ.vi"("in Rotation3d"=w501) -> ("Z"=w493:dbl, "Y"=w494:dbl, "X"=w495:dbl)  [unwired: 8 in]
  n140 = call <vilib>:"Rotation3d_Equals.vi"("other Rotation3d"=w576, "in Rotation3d"=w577) -> ("Equals"=w565:bool)  [unwired: 9 in]
  n141 = call <vilib>:"Rotation3d_Minus.vi"("other Rotation3d"=w329, "in Rotation3d"=w322) -> ("out Rotation3d"=w330:T1)  [unwired: 9 in]
  n142 = call <vilib>:"Conv_Deg_Radians.vi"("Degress"=90.0) -> ("Radians"=w272:dbl)  [unwired: 10 in]
  n143 = call <vilib>:"Conv_Deg_Radians.vi"("Degress"=45.0) -> ("Radians"=w261:dbl)  [unwired: 10 in]
  n144 = call <vilib>:"Conv_Deg_Radians.vi"("Degress"=60.0) -> ("Radians"=w254:dbl)  [unwired: 10 in]
  n145 = call <vilib>:"Rotation3d_Equals.vi"("other Rotation3d"=w567, "in Rotation3d"=w568) -> ("Equals"=w564:bool)  [unwired: 9 in]
  n146 = call <vilib>:"Rotation3d_Equals.vi"("other Rotation3d"=w475, "in Rotation3d"=w468) -> ("Equals"=w474:bool)  [unwired: 9 in]
  n147 = call <vilib>:"Rotation3d_Equals.vi"("other Rotation3d"=w464, "in Rotation3d"=w454) -> ("Equals"=w458:bool)  [unwired: 9 in]
  n148 = call <vilib>:"Rotation3d_Equals.vi"("other Rotation3d"=w407, "in Rotation3d"=w409) -> ("Equals"=w406:bool)  [unwired: 9 in]
  n149 = call <vilib>:"Rotation3d_Equals.vi"("other Rotation3d"=w417, "in Rotation3d"=w419) -> ("Equals"=w416:bool)  [unwired: 9 in]
  n150 = call <vilib>:"Rotation3d_Equals.vi"("other Rotation3d"=w427, "in Rotation3d"=w428) -> ("Equals"=w426:bool)  [unwired: 9 in]
  n151 = call <vilib>:"Rotation3d_Equals.vi"("other Rotation3d"=w384, "in Rotation3d"=w399) -> ("Equals"=w383:bool)  [unwired: 9 in]
  n152 = call <vilib>:"Rotation3d_Equals.vi"("other Rotation3d"=w361, "in Rotation3d"=w376) -> ("Equals"=w360:bool)  [unwired: 9 in]
  n153 = call <vilib>:"Rotation3d_ToRotation2d.vi"("in Rotation3d"=w227) -> ("out Rotation2d"=w226:T3)  [unwired: 10 in]
  n154 = call <vilib>:"Rotation3d_Equals.vi"("other Rotation3d"=w438, "in Rotation3d"=w439) -> ("Equals"=w437:bool)  [unwired: 9 in]
  n155 = call <vilib>:"Rotation3d_Equals.vi"("other Rotation3d"=w447, "in Rotation3d"=w442) -> ("Equals"=w446:bool)  [unwired: 9 in]
  n156 = call <vilib>:"Rotation3d_Equals.vi"("other Rotation3d"=w338, "in Rotation3d"=w353) -> ("Equals"=w337:bool)  [unwired: 9 in]
  n157 = call <vilib>:"Rotation3d_Equals.vi"("other Rotation3d"=w210, "in Rotation3d"=w211) -> ("Equals"=w209:bool)  [unwired: 9 in]
  n158 = call <vilib>:"Rotation3d_Equals.vi"("other Rotation3d"=w315, "in Rotation3d"=w330) -> ("Equals"=w314:bool)  [unwired: 9 in]
  n159 = call <vilib>:"Rotation3d_Equals.vi"("other Rotation3d"=w301, "in Rotation3d"=w300) -> ("Equals"=w285:bool)  [unwired: 9 in]
  n160 = call <vilib>:"Conv_Deg_Radians.vi"("Degress"=50.0) -> ("Radians"=w197:dbl)  [unwired: 10 in]
  n161 = call <vilib>:"Conv_Deg_Radians.vi"("Degress"=70.0) -> ("Radians"=w195:dbl)  [unwired: 10 in]
  n162 = call <vilib>:"Rotation3d_Equals.vi"("other Rotation3d"=w287, "in Rotation3d"=w286) -> ("Equals"=w284:bool)  [unwired: 9 in]
  n163 = call <vilib>:"Conv_Deg_Radians.vi"("Degress"=170.0) -> ("Radians"=w167:dbl)  [unwired: 10 in]
  n164 = call <vilib>:"Conv_Deg_Radians.vi"("Degress"=-160.0) -> ("Radians"=w165:dbl)  [unwired: 10 in]
  n165 = call <vilib>:"Conv_Deg_Radians.vi"("Degress"=50.0) -> ("Radians"=w136:dbl)  [unwired: 10 in]
  n166 = call <vilib>:"Conv_Deg_Radians.vi"("Degress"=70.0) -> ("Radians"=w134:dbl)  [unwired: 10 in]
  n167 = call <vilib>:"Rotation3d_Create_AxisAngle.vi"("Angle"=w272, "Axis Vector"=w269) -> ("Rotation3d"=w271:T1)  [unwired: 9 in]
  n168 = call <vilib>:"Conv_Deg_Radians.vi"("Degress"=170.0) -> ("Radians"=w111:dbl)  [unwired: 10 in]
  n169 = call <vilib>:"Conv_Deg_Radians.vi"("Degress"=-160.0) -> ("Radians"=w109:dbl)  [unwired: 10 in]
  n170 = call <vilib>:"Rotation3d_Create_AxisAngle.vi"("Angle"=w261, "Axis Vector"=w248) -> ("Rotation3d"=w260:T1)  [unwired: 9 in]
  n171 = call <vilib>:"Rotation3d_Create_AxisAngle.vi"("Angle"=w254, "Axis Vector"=w247) -> ("Rotation3d"=w253:T1)  [unwired: 9 in]
  n172 = call <vilib>:"Conv_Deg_Radians.vi"("Degress"=50.0) -> ("Radians"=w71:dbl)  [unwired: 10 in]
  n173 = call <vilib>:"Conv_Deg_Radians.vi"("Degress"=70.0) -> ("Radians"=w69:dbl)  [unwired: 10 in]
  n174 = call <vilib>:"Conv_Deg_Radians.vi"("Degress"=170.0) -> ("Radians"=w46:dbl)  [unwired: 10 in]
  n175 = call <vilib>:"Conv_Deg_Radians.vi"("Degress"=-160.0) -> ("Radians"=w44:dbl)  [unwired: 10 in]
  n176 = call <vilib>:"Util_ApproxEquals.vi"("Value 2"=0.0, "Value 1"=w544) -> ("ApproxEquals"=w547:bool)  [unwired: 9 in]
  n177 = call <vilib>:"Util_ApproxEquals.vi"("Value 2"=w541, "Value 1"=w543) -> ("ApproxEquals"=w546:bool)  [unwired: 9 in]
  n178 = call <vilib>:"Util_ApproxEquals.vi"("Value 2"=0.0, "Value 1"=w545) -> ("ApproxEquals"=w548:bool)  [unwired: 9 in]
  n179 = Compound Arithmetic op=AND(w566, w565, w564) -> (w563:bool)
  n180 = call <vilib>:"Util_ApproxEquals.vi"("Value 2"=0.0, "Value 1"=w525) -> ("ApproxEquals"=w528:bool)  [unwired: 9 in]
  n181 = call <vilib>:"Util_ApproxEquals.vi"("Value 2"=w522, "Value 1"=w524) -> ("ApproxEquals"=w527:bool)  [unwired: 9 in]
  n182 = call <vilib>:"Util_ApproxEquals.vi"("Value 2"=0.0, "Value 1"=w508) -> ("ApproxEquals"=w511:bool)  [unwired: 9 in]
  n183 = call <vilib>:"Util_ApproxEquals.vi"("Value 2"=w487, "Value 1"=w507) -> ("ApproxEquals"=w510:bool)  [unwired: 9 in]
  n184 = call <vilib>:"Util_ApproxEquals.vi"("Value 2"=0.0, "Value 1"=w526) -> ("ApproxEquals"=w529:bool)  [unwired: 9 in]
  n185 = call <vilib>:"Util_ApproxEquals.vi"("Value 2"=0.0, "Value 1"=w509) -> ("ApproxEquals"=w512:bool)  [unwired: 9 in]
  n186 = call <vilib>:"Util_ApproxEquals.vi"("Value 2"=0.0, "Value 1"=w494) -> ("ApproxEquals"=w497:bool)  [unwired: 9 in]
  n187 = call <vilib>:"Util_ApproxEquals.vi"("Value 2"=w482, "Value 1"=w493) -> ("ApproxEquals"=w496:bool)  [unwired: 9 in]
  n188 = call <vilib>:"Util_ApproxEquals.vi"("Value 2"=0.0, "Value 1"=w495) -> ("ApproxEquals"=w498:bool)  [unwired: 9 in]
  n189 = call <vilib>:"Rotation3d_Create_AxisAngle.vi"("Angle"=w197, "Axis Vector"=w140) -> ("Rotation3d"=w191:T1)  [unwired: 9 in]
  n190 = call <vilib>:"Rotation3d_Create_AxisAngle.vi"("Angle"=w195, "Axis Vector"=w140) -> ("Rotation3d"=w190:T1)  [unwired: 9 in]
  n191 = call <vilib>:"Rotation3d_Create_AxisAngle.vi"("Angle"=w167, "Axis Vector"=w140) -> ("Rotation3d"=w161:T1)  [unwired: 9 in]
  n192 = call <vilib>:"Rotation3d_Create_AxisAngle.vi"("Angle"=w165, "Axis Vector"=w140) -> ("Rotation3d"=w160:T1)  [unwired: 9 in]
  n193 = call <vilib>:"Rotation2d_Equals.vi"("other ROTATION"=w225, "in ROTATION"=w226) -> ("Equals"=w224:bool)  [unwired: 9 in]
  n194 = call <vilib>:"Rotation3d_Create_AxisAngle.vi"("Angle"=w136, "Axis Vector"=w89) -> ("Rotation3d"=w130:T1)  [unwired: 9 in]
  n195 = call <vilib>:"Rotation3d_Create_AxisAngle.vi"("Angle"=w134, "Axis Vector"=w89) -> ("Rotation3d"=w129:T1)  [unwired: 9 in]
  n196 = Not(x=w209) -> (.not. x?=w208:bool)
  n197 = call <vilib>:"Rotation3d_Create_AxisAngle.vi"("Angle"=w111, "Axis Vector"=w89) -> ("Rotation3d"=w105:T1)  [unwired: 9 in]
  n198 = call <vilib>:"Rotation3d_Create_AxisAngle.vi"("Angle"=w109, "Axis Vector"=w89) -> ("Rotation3d"=w104:T1)  [unwired: 9 in]
  n199 = call <vilib>:"Rotation3d_GetAxisAngle.vi"("in Rotation3d"=w271) -> ("Angle"=w266:dbl, "Axis Vector"=w270:dbl[])  [unwired: 9 in]
  n200 = call <vilib>:"Rotation3d_GetAxisAngle.vi"("in Rotation3d"=w260) -> ("Angle"=w256:dbl, "Axis Vector"=w259:dbl[])  [unwired: 9 in]
  n201 = call <vilib>:"Rotation3d_Create_AxisAngle.vi"("Angle"=w71, "Axis Vector"=w12) -> ("Rotation3d"=w65:T1)  [unwired: 9 in]
  n202 = call <vilib>:"Rotation3d_Create_AxisAngle.vi"("Angle"=w69, "Axis Vector"=w12) -> ("Rotation3d"=w64:T1)  [unwired: 9 in]
  n203 = call <vilib>:"Rotation3d_GetAxisAngle.vi"("in Rotation3d"=w253) -> ("Angle"=w249:dbl, "Axis Vector"=w252:dbl[])  [unwired: 9 in]
  n204 = call <vilib>:"Rotation3d_Create_AxisAngle.vi"("Angle"=w46, "Axis Vector"=w12) -> ("Rotation3d"=w40:T1)  [unwired: 9 in]
  n205 = call <vilib>:"Rotation3d_Create_AxisAngle.vi"("Angle"=w44, "Axis Vector"=w12) -> ("Rotation3d"=w39:T1)  [unwired: 9 in]
  n206 = Compound Arithmetic op=AND(w285, w284) -> (w283:bool)
  n207 = Multiply(x=1.5707963267948966, y=0.5) -> (x*y=w244:dbl)
  n208 = call-poly <vilib>:"Array To Matrix.vi"("Real 1D Array"=w269) -> ("Real Matrix (Column Vector)"=w268:T4)
  n209 = call-poly <vilib>:"Array To Matrix.vi"("Real 1D Array"=w248) -> ("Real Matrix (Column Vector)"=w258:T4)
  n210 = call-poly <vilib>:"Array To Matrix.vi"("Real 1D Array"=w270) -> ("Real Matrix (Column Vector)"=w267:T4)
  n211 = call-poly <vilib>:"Array To Matrix.vi"("Real 1D Array"=w259) -> ("Real Matrix (Column Vector)"=w257:T4)
  n212 = call-poly <vilib>:"Array To Matrix.vi"("Real 1D Array"=w247) -> ("Real Matrix (Column Vector)"=w251:T4)
  n213 = call-poly <vilib>:"Array To Matrix.vi"("Real 1D Array"=w252) -> ("Real Matrix (Column Vector)"=w250:T4)
  n214 = Divide(x=3.141592653589793, y=3.0) -> (x/y=w239:dbl)
  n215 = Compound Arithmetic op=AND(w548, w547, w546) -> (w540:bool)
  n216 = Compound Arithmetic op=AND(w529, w528, w527) -> (w521:bool)
  n217 = Compound Arithmetic op=AND(w512, w511, w510) -> (w506:bool)
  n218 = Compound Arithmetic op=AND(w498, w497, w496) -> (w492:bool)
  n219 = call <vilib>:"Util_ApproxEquals.vi"("Value 2"=1.5707963267948966, "Value 1"=w266) -> ("ApproxEquals"=w263:bool)  [unwired: 9 in]
  n220 = call <vilib>:"Matrix_IsEqual.vi"("other"=w267, "input matrix"=w268) -> ("Equal"=w264:bool)  [unwired: 9 in]
  n221 = call <vilib>:"Util_ApproxEquals.vi"("Value 2"=w244, "Value 1"=w256) -> ("ApproxEquals"=w242:bool)  [unwired: 9 in]
  n222 = call <vilib>:"Matrix_IsEqual.vi"("other"=w257, "input matrix"=w258) -> ("Equal"=w243:bool)  [unwired: 9 in]
  n223 = call <vilib>:"Util_ApproxEquals.vi"("Value 2"=w239, "Value 1"=w249) -> ("ApproxEquals"=w237:bool)  [unwired: 9 in]
  n224 = call <vilib>:"Matrix_IsEqual.vi"("other"=w250, "input matrix"=w251) -> ("Equal"=w238:bool)  [unwired: 9 in]
  n225 = Compound Arithmetic op=AND(w474, w458, w446, w437) -> (w436:bool)
  n226 = call <vilib>:"Rotation3d_Interpolate.vi"("T"=0.25, "EndValue Rotation3d"=w190, "in Rotation3d"=w191) -> ("Interpolated Rotation3d"=w178:T1)  [unwired: 8 in]
  n227 = call <vilib>:"Rotation3d_Interpolate.vi"("T"=0.5, "EndValue Rotation3d"=w190, "in Rotation3d"=w191) -> ("Interpolated Rotation3d"=w181:T1)  [unwired: 8 in]
  n228 = call <vilib>:"Rotation3d_Interpolate.vi"("T"=0.25, "EndValue Rotation3d"=w160, "in Rotation3d"=w161) -> ("Interpolated Rotation3d"=w148:T1)  [unwired: 8 in]
  n229 = call <vilib>:"Rotation3d_Interpolate.vi"("T"=0.75, "EndValue Rotation3d"=w190, "in Rotation3d"=w191) -> ("Interpolated Rotation3d"=w175:T1)  [unwired: 8 in]
  n230 = call <vilib>:"Rotation3d_Interpolate.vi"("T"=0.5, "EndValue Rotation3d"=w160, "in Rotation3d"=w161) -> ("Interpolated Rotation3d"=w151:T1)  [unwired: 8 in]
  n231 = call <vilib>:"Rotation3d_Interpolate.vi"("T"=0.25, "EndValue Rotation3d"=w129, "in Rotation3d"=w130) -> ("Interpolated Rotation3d"=w118:T1)  [unwired: 8 in]
  n232 = call <vilib>:"Rotation3d_Interpolate.vi"("T"=0.75, "EndValue Rotation3d"=w160, "in Rotation3d"=w161) -> ("Interpolated Rotation3d"=w145:T1)  [unwired: 8 in]
  n233 = call <vilib>:"Rotation3d_Interpolate.vi"("T"=0.5, "EndValue Rotation3d"=w129, "in Rotation3d"=w130) -> ("Interpolated Rotation3d"=w121:T1)  [unwired: 8 in]
  n234 = call <vilib>:"Rotation3d_Interpolate.vi"("T"=0.25, "EndValue Rotation3d"=w104, "in Rotation3d"=w105) -> ("Interpolated Rotation3d"=w96:T1)  [unwired: 8 in]
  n235 = call <vilib>:"Rotation3d_Interpolate.vi"("T"=0.75, "EndValue Rotation3d"=w129, "in Rotation3d"=w130) -> ("Interpolated Rotation3d"=w115:T1)  [unwired: 8 in]
  n236 = call <vilib>:"Rotation3d_Interpolate.vi"("T"=0.5, "EndValue Rotation3d"=w104, "in Rotation3d"=w105) -> ("Interpolated Rotation3d"=w98:T1)  [unwired: 8 in]
  n237 = call <vilib>:"Rotation3d_Interpolate.vi"("T"=0.75, "EndValue Rotation3d"=w104, "in Rotation3d"=w105) -> ("Interpolated Rotation3d"=w93:T1)  [unwired: 8 in]
  n238 = call <vilib>:"Rotation3d_Interpolate.vi"("T"=0.25, "EndValue Rotation3d"=w64, "in Rotation3d"=w65) -> ("Interpolated Rotation3d"=w53:T1)  [unwired: 8 in]
  n239 = call <vilib>:"Rotation3d_Interpolate.vi"("T"=0.5, "EndValue Rotation3d"=w64, "in Rotation3d"=w65) -> ("Interpolated Rotation3d"=w56:T1)  [unwired: 8 in]
  n240 = call <vilib>:"Rotation3d_Interpolate.vi"("T"=0.25, "EndValue Rotation3d"=w39, "in Rotation3d"=w40) -> ("Interpolated Rotation3d"=w31:T1)  [unwired: 8 in]
  n241 = call <vilib>:"Rotation3d_Interpolate.vi"("T"=0.75, "EndValue Rotation3d"=w64, "in Rotation3d"=w65) -> ("Interpolated Rotation3d"=w50:T1)  [unwired: 8 in]
  n242 = call <vilib>:"Rotation3d_Interpolate.vi"("T"=0.5, "EndValue Rotation3d"=w39, "in Rotation3d"=w40) -> ("Interpolated Rotation3d"=w33:T1)  [unwired: 8 in]
  n243 = call <vilib>:"Rotation3d_Interpolate.vi"("T"=0.75, "EndValue Rotation3d"=w39, "in Rotation3d"=w40) -> ("Interpolated Rotation3d"=w28:T1)  [unwired: 8 in]
  n244 = Compound Arithmetic op=AND(w540, w521) -> (w520:bool)
  n245 = Compound Arithmetic op=AND(w506, w492) -> (w481:bool)
  n246 = Compound Arithmetic op=AND(w264, w263, w243, w242, w238, w237) -> (w236:bool)
  n247 = call <vilib>:"Rotation3d_GetXYZ.vi"("in Rotation3d"=w178) -> ("X"=w174:dbl)  [unwired: 8 in, 2 out]
  n248 = call <vilib>:"Conv_Deg_Radians.vi"("Degress"=55.0) -> ("Radians"=w179:dbl)  [unwired: 10 in]
  n249 = call <vilib>:"Rotation3d_GetXYZ.vi"("in Rotation3d"=w181) -> ("Z"=w183:dbl, "Y"=w184:dbl, "X"=w185:dbl)  [unwired: 8 in]
  n250 = call <vilib>:"Rotation3d_GetXYZ.vi"("in Rotation3d"=w148) -> ("X"=w139:dbl)  [unwired: 8 in, 2 out]
  n251 = call <vilib>:"Conv_Deg_Radians.vi"("Degress"=177.5) -> ("Radians"=w149:dbl)  [unwired: 10 in]
  n252 = call <vilib>:"Rotation3d_GetXYZ.vi"("in Rotation3d"=w175) -> ("X"=w171:dbl)  [unwired: 8 in, 2 out]
  n253 = call <vilib>:"Conv_Deg_Radians.vi"("Degress"=65.0) -> ("Radians"=w176:dbl)  [unwired: 10 in]
  n254 = call <vilib>:"Conv_Deg_Radians.vi"("Degress"=60.0) -> ("Radians"=w172:dbl)  [unwired: 10 in]
  n255 = call <vilib>:"Rotation3d_GetXYZ.vi"("in Rotation3d"=w151) -> ("Z"=w153:dbl, "Y"=w154:dbl, "X"=w155:dbl)  [unwired: 8 in]
  n256 = call <vilib>:"Rotation3d_GetXYZ.vi"("in Rotation3d"=w118) -> ("Y"=w92:dbl)  [unwired: 8 in, 2 out]
  n257 = call <vilib>:"Conv_Deg_Radians.vi"("Degress"=55.0) -> ("Radians"=w119:dbl)  [unwired: 10 in]
  n258 = call <vilib>:"Rotation3d_GetXYZ.vi"("in Rotation3d"=w145) -> ("X"=w138:dbl)  [unwired: 8 in, 2 out]
  n259 = call <vilib>:"Conv_Deg_Radians.vi"("Degress"=-167.5) -> ("Radians"=w146:dbl)  [unwired: 10 in]
  n260 = call <vilib>:"Conv_Deg_Radians.vi"("Degress"=-175.0) -> ("Radians"=w143:dbl)  [unwired: 10 in]
  n261 = call <vilib>:"Rotation3d_GetXYZ.vi"("in Rotation3d"=w121) -> ("Z"=w123:dbl, "Y"=w124:dbl, "X"=w125:dbl)  [unwired: 8 in]
  n262 = call <vilib>:"Rotation3d_GetXYZ.vi"("in Rotation3d"=w96) -> ("Y"=w75:dbl)  [unwired: 8 in, 2 out]
  n263 = call <vilib>:"Conv_Deg_Radians.vi"("Degress"=2.5) -> ("Radians"=w76:dbl)  [unwired: 10 in]
  n264 = call <vilib>:"Rotation3d_GetXYZ.vi"("in Rotation3d"=w115) -> ("Y"=w91:dbl)  [unwired: 8 in, 2 out]
  n265 = call <vilib>:"Conv_Deg_Radians.vi"("Degress"=65.0) -> ("Radians"=w116:dbl)  [unwired: 10 in]
  n266 = call <vilib>:"Conv_Deg_Radians.vi"("Degress"=0.0) -> ("Radians"=w83:dbl)  [unwired: 10 in]
  n267 = call <vilib>:"Conv_Deg_Radians.vi"("Degress"=60.0) -> ("Radians"=w84:dbl)  [unwired: 10 in]
  n268 = call <vilib>:"Conv_Deg_Radians.vi"("Degress"=0.0) -> ("Radians"=w85:dbl)  [unwired: 10 in]
  n269 = call <vilib>:"Rotation3d_GetXYZ.vi"("in Rotation3d"=w98) -> ("Z"=w99:dbl, "Y"=w88:dbl, "X"=w100:dbl)  [unwired: 8 in]
  n270 = call <vilib>:"Conv_Deg_Radians.vi"("Degress"=180.0) -> ("Radians"=w79:dbl)  [unwired: 10 in]
  n271 = call <vilib>:"Conv_Deg_Radians.vi"("Degress"=-5.0) -> ("Radians"=w78:dbl)  [unwired: 10 in]
  n272 = call <vilib>:"Conv_Deg_Radians.vi"("Degress"=180.0) -> ("Radians"=w77:dbl)  [unwired: 10 in]
  n273 = call <vilib>:"Rotation3d_GetXYZ.vi"("in Rotation3d"=w93) -> ("Y"=w90:dbl)  [unwired: 8 in, 2 out]
  n274 = call <vilib>:"Conv_Deg_Radians.vi"("Degress"=-12.5) -> ("Radians"=w94:dbl)  [unwired: 10 in]
  n275 = call <vilib>:"Rotation3d_GetXYZ.vi"("in Rotation3d"=w53) -> ("Z"=w11:dbl)  [unwired: 8 in, 2 out]
  n276 = call <vilib>:"Conv_Deg_Radians.vi"("Degress"=55.0) -> ("Radians"=w54:dbl)  [unwired: 10 in]
  n277 = call <vilib>:"Rotation3d_GetXYZ.vi"("in Rotation3d"=w56) -> ("Z"=w58:dbl, "Y"=w59:dbl, "X"=w60:dbl)  [unwired: 8 in]
  n278 = call <vilib>:"Rotation3d_GetXYZ.vi"("in Rotation3d"=w31) -> ("Z"=w9:dbl)  [unwired: 8 in, 2 out]
  n279 = call <vilib>:"Conv_Deg_Radians.vi"("Degress"=177.5) -> ("Radians"=w15:dbl)  [unwired: 10 in]
  n280 = call <vilib>:"Rotation3d_GetXYZ.vi"("in Rotation3d"=w50) -> ("Z"=w10:dbl)  [unwired: 8 in, 2 out]
  n281 = call <vilib>:"Conv_Deg_Radians.vi"("Degress"=65.0) -> ("Radians"=w51:dbl)  [unwired: 10 in]
  n282 = call <vilib>:"Conv_Deg_Radians.vi"("Degress"=0.0) -> ("Radians"=w22:dbl)  [unwired: 10 in]
  n283 = call <vilib>:"Conv_Deg_Radians.vi"("Degress"=0.0) -> ("Radians"=w23:dbl)  [unwired: 10 in]
  n284 = call <vilib>:"Conv_Deg_Radians.vi"("Degress"=60.0) -> ("Radians"=w24:dbl)  [unwired: 10 in]
  n285 = call <vilib>:"Rotation3d_GetXYZ.vi"("in Rotation3d"=w33) -> ("Z"=w34:dbl, "Y"=w27:dbl, "X"=w35:dbl)  [unwired: 8 in]
  n286 = call <vilib>:"Conv_Deg_Radians.vi"("Degress"=0.0) -> ("Radians"=w18:dbl)  [unwired: 10 in]
  n287 = call <vilib>:"Conv_Deg_Radians.vi"("Degress"=0.0) -> ("Radians"=w17:dbl)  [unwired: 10 in]
  n288 = call <vilib>:"Conv_Deg_Radians.vi"("Degress"=-175.0) -> ("Radians"=w16:dbl)  [unwired: 10 in]
  n289 = call <vilib>:"Rotation3d_GetXYZ.vi"("in Rotation3d"=w28) -> ("Z"=w8:dbl)  [unwired: 8 in, 2 out]
  n290 = call <vilib>:"Conv_Deg_Radians.vi"("Degress"=-167.5) -> ("Radians"=w29:dbl)  [unwired: 10 in]
  n291 = call <vilib>:"Util_ApproxEquals.vi"("Value 2"=w179, "Value 1"=w174) -> ("ApproxEquals"=w170:bool)  [unwired: 9 in]
  n292 = call <vilib>:"Util_ApproxEquals.vi"("Value 2"=w149, "Value 1"=w139) -> ("ApproxEquals"=w142:bool)  [unwired: 9 in]
  n293 = call <vilib>:"Util_ApproxEquals.vi"("Value 2"=0.0, "Value 1"=w184) -> ("ApproxEquals"=w187:bool)  [unwired: 9 in]
  n294 = call <vilib>:"Util_ApproxEquals.vi"("Value 2"=0.0, "Value 1"=w183) -> ("ApproxEquals"=w186:bool)  [unwired: 9 in]
  n295 = call <vilib>:"Util_ApproxEquals.vi"("Value 2"=w172, "Value 1"=w185) -> ("ApproxEquals"=w188:bool)  [unwired: 9 in]
  n296 = call <vilib>:"Util_ApproxEquals.vi"("Value 2"=w176, "Value 1"=w171) -> ("ApproxEquals"=w169:bool)  [unwired: 9 in]
  n297 = call <vilib>:"Util_ApproxEquals.vi"("Value 2"=w119, "Value 1"=w92) -> ("ApproxEquals"=w114:bool)  [unwired: 9 in]
  n298 = call <vilib>:"Util_ApproxEquals.vi"("Value 2"=0.0, "Value 1"=w154) -> ("ApproxEquals"=w157:bool)  [unwired: 9 in]
  n299 = call <vilib>:"Util_ApproxEquals.vi"("Value 2"=0.0, "Value 1"=w153) -> ("ApproxEquals"=w156:bool)  [unwired: 9 in]
  n300 = call <vilib>:"Util_ApproxEquals.vi"("Value 2"=w143, "Value 1"=w155) -> ("ApproxEquals"=w158:bool)  [unwired: 9 in]
  n301 = call <vilib>:"Util_ApproxEquals.vi"("Value 2"=w146, "Value 1"=w138) -> ("ApproxEquals"=w141:bool)  [unwired: 9 in]
  n302 = call <vilib>:"Util_ApproxEquals.vi"("Value 2"=w76, "Value 1"=w75) -> ("ApproxEquals"=w74:bool)  [unwired: 9 in]
  n303 = call <vilib>:"Util_ApproxEquals.vi"("Value 2"=w84, "Value 1"=w124) -> ("ApproxEquals"=w127:bool)  [unwired: 9 in]
  n304 = call <vilib>:"Util_ApproxEquals.vi"("Value 2"=w85, "Value 1"=w123) -> ("ApproxEquals"=w126:bool)  [unwired: 9 in]
  n305 = call <vilib>:"Util_ApproxEquals.vi"("Value 2"=w83, "Value 1"=w125) -> ("ApproxEquals"=w128:bool)  [unwired: 9 in]
  n306 = call <vilib>:"Util_ApproxEquals.vi"("Value 2"=w116, "Value 1"=w91) -> ("ApproxEquals"=w113:bool)  [unwired: 9 in]
  n307 = call <vilib>:"Util_ApproxEquals.vi"("Value 2"=w78, "Value 1"=w88) -> ("ApproxEquals"=w102:bool)  [unwired: 9 in]
  n308 = call <vilib>:"Util_ApproxEquals.vi"("Value 2"=w77, "Value 1"=w99) -> ("ApproxEquals"=w101:bool)  [unwired: 9 in]
  n309 = call <vilib>:"Util_ApproxEquals.vi"("Value 2"=w79, "Value 1"=w100) -> ("ApproxEquals"=w103:bool)  [unwired: 9 in]
  n310 = call <vilib>:"Util_ApproxEquals.vi"("Value 2"=w94, "Value 1"=w90) -> ("ApproxEquals"=w73:bool)  [unwired: 9 in]
  n311 = call <vilib>:"Util_ApproxEquals.vi"("Value 2"=w54, "Value 1"=w11) -> ("ApproxEquals"=w49:bool)  [unwired: 9 in]
  n312 = call <vilib>:"Util_ApproxEquals.vi"("Value 2"=w15, "Value 1"=w9) -> ("ApproxEquals"=w14:bool)  [unwired: 9 in]
  n313 = call <vilib>:"Util_ApproxEquals.vi"("Value 2"=w23, "Value 1"=w59) -> ("ApproxEquals"=w62:bool)  [unwired: 9 in]
  n314 = call <vilib>:"Util_ApproxEquals.vi"("Value 2"=w24, "Value 1"=w58) -> ("ApproxEquals"=w61:bool)  [unwired: 9 in]
  n315 = call <vilib>:"Util_ApproxEquals.vi"("Value 2"=w22, "Value 1"=w60) -> ("ApproxEquals"=w63:bool)  [unwired: 9 in]
  n316 = call <vilib>:"Util_ApproxEquals.vi"("Value 2"=w51, "Value 1"=w10) -> ("ApproxEquals"=w48:bool)  [unwired: 9 in]
  n317 = call <vilib>:"Util_ApproxEquals.vi"("Value 2"=w17, "Value 1"=w27) -> ("ApproxEquals"=w37:bool)  [unwired: 9 in]
  n318 = call <vilib>:"Util_ApproxEquals.vi"("Value 2"=w16, "Value 1"=w34) -> ("ApproxEquals"=w36:bool)  [unwired: 9 in]
  n319 = call <vilib>:"Util_ApproxEquals.vi"("Value 2"=w18, "Value 1"=w35) -> ("ApproxEquals"=w38:bool)  [unwired: 9 in]
  n320 = call <vilib>:"Util_ApproxEquals.vi"("Value 2"=w29, "Value 1"=w8) -> ("ApproxEquals"=w13:bool)  [unwired: 9 in]
  n321 = Compound Arithmetic op=AND(w170, w188, w187, w186, w169) -> (w7:bool)
  n322 = Compound Arithmetic op=AND(w142, w158, w157, w156, w141) -> (w6:bool)
  n323 = Compound Arithmetic op=AND(w114, w128, w127, w126, w113) -> (w5:bool)
  n324 = Compound Arithmetic op=AND(w74, w103, w102, w101, w73) -> (w4:bool)
  n325 = Compound Arithmetic op=AND(w49, w63, w62, w61, w48) -> (w3:bool)
  n326 = Compound Arithmetic op=AND(w14, w38, w37, w36, w13) -> (w2:bool)
  n327 = Compound Arithmetic op=AND(w7, w6, w5, w4, w3, w2) -> (w1:bool)
  n328 = Compound Arithmetic op=AND(w563, w520, w481, w436, w426, w416, w406, w383, w360, w337, w314, w283, w236, w224, w208, w1) -> (→"ALL TESTS PASSED":bool)
  "error out" <- "error in (no error)"
